vi "Initialize.vi"(0 "NI Build Specification_LV in":refnum<class "NI Build Specification_LV.lvclass">) -> (4 "NI Build Specification_LV out":refnum<class "NI Build Specification_LV.lvclass">)   [LabVIEW 2017, in "CL_G3_VIComponentBuilder.lvlib" / "NI Build Specification_LV.lvclass"]
doc: "Responsible for determining the Unique Name, Product Name, and Export's Build Specification file."
uses:
  NI Build Specification_LV.lvclass
  C:/builds/Component BuilderBT/SrcDist/Exports/Exports/Export.lvclass
  Exports/Export.lvclass/Export.ctl
  NI Build Specification_LV.lvclass/NI Build Specification_LV.ctl
  Accessors/Read Display Name XML Prop Name.vi
  Accessors/Read Unique Name XML Prop Name.vi
  Exports/Accessors/Write Export Operation Errors.vi
  Exports/Accessors/Read Export Build Specification.vi
  <vilib>/xml/Close Reference(Node).vi
  Exports/Accessors/Write Product Name.vi
  Exports/Accessors/Write unique Name.vi
  Exports/Export.lvclass
  <resource>/objmgr/DOMUserDefRef.rc
  <vilib>/xml/NI_XML.lvlib
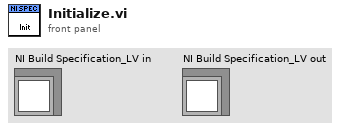
[diagram p1: front panel]
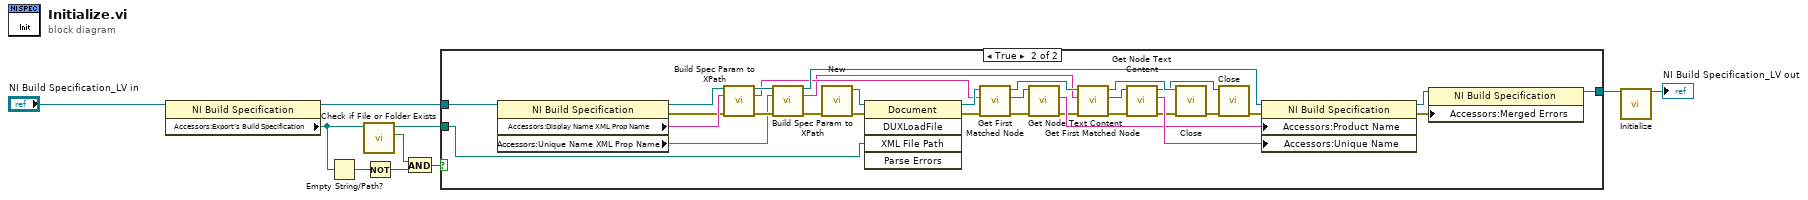
[diagram p0: block diagram]
diagram:
  n1 = property class="NI Build Specification"(reference="NI Build Specification_LV in") -> (reference out=w9:refnum<class "NI Build Specification_LV.lvclass">, "Accessors:Export's Build Specification"=w3:path)  [unwired: 1 in, 1 out]
  n2 = Empty String/Path?(string/path=w3) -> (empty?=w8:bool)
  n3 = call <vilib>:"Check if File or Folder Exists.vi"("path"=w3) -> ("file or folder exists?"=w7:bool, "dup path"=w5:path)  [unwired: 8 in, 1 out]
  n4 = Not(x=w8) -> (.not. x?=w6:bool)
  n5 = And(x=w7, y=w6) -> (x .and. y?=w4:bool)
  n6 = case shown="True" w4 {
    tunnel: w9 -> [w11 w25]
    tunnel: [w11 w40] -> w2
    tunnel: w5 -> [_ w38]
    frame False {
    }
    frame True {
      n7 = property class="NI Build Specification"(reference=w25) -> (reference out=w24:refnum<class "NI Build Specification_LV.lvclass">, error out=w13:errorcluster, "Accessors:Display Name XML Prop Name"=w20:string, "Accessors:Unique Name XML Prop Name"=w19:string)  [unwired: 1 in]
      n8 = call-dynamic "Build Spec Param to XPath.vi"("NI Build Specification"=w24, "Build Spec Parameter Name"=w20, "error in (no error)"=w13) -> ("NI Build Specification"=w23:refnum<class "NI Build Specification_LV.lvclass">, "XPath to the specific build Spec Property"=w18:string, "error out"=w21:errorcluster)  [unwired: 10 in]
      n9 = call-dynamic "Build Spec Param to XPath.vi"("NI Build Specification"=w23, "Build Spec Parameter Name"=w19, "error in (no error)"=w21) -> ("NI Build Specification"=w22:refnum<class "NI Build Specification_LV.lvclass">, "XPath to the specific build Spec Property"=w17:string, "error out"=w12:errorcluster)  [unwired: 10 in]
      n10 = call <vilib>:"New.vi"("error in (no error)"=w12) -> ("error out"=w27:errorcluster, "DOM document out"=w26:refnum<k20>)  [unwired: 7 in]
      n11 = invoke class="Document" method="DUXLoadFile"(reference=w26, error in=w27, "XML File Path"=w38) -> (reference out=w28:refnum<k20>, error out=w30:errorcluster)  [unwired: 2 in, 3 out]
      n12 = call <vilib>:"Get First Matched Node.vi"("error in (no error)"=w30, "XPath expression"=w18, "node in"=w28) -> ("error out"=w31:errorcluster, "node result"=w29:refnum<k20>, "node out"=w34:refnum<k20>)  [unwired: 6 in]
      n13 = call <vilib>:"Get Node Text Content.vi"("error in (no error)"=w31, "node in"=w29) -> ("error out"=w33:errorcluster, "node text"=w41:string)  [unwired: 7 in, 1 out]
      n14 = call <vilib>:"Get First Matched Node.vi"("error in (no error)"=w33, "XPath expression"=w17, "node in"=w34) -> ("error out"=w32:errorcluster, "node result"=w35:refnum<k20>, "node out"=w36:refnum<k20>)  [unwired: 6 in]
      n15 = call <vilib>:"Get Node Text Content.vi"("error in (no error)"=w32, "node in"=w35) -> ("error out"=w37:errorcluster, "node text"=w42:string, "node out"=w16:refnum<k20>)  [unwired: 7 in]
      n16 = call-poly <vilib>:"Close.vi"("error in (no error)"=w37, "node"=w36) -> ("error out"=w15:errorcluster)  [unwired: 7 in]
      n17 = call-poly <vilib>:"Close.vi"("error in (no error)"=w15, "node"=w16) -> ("error out"=w14:errorcluster)  [unwired: 7 in]
      n18 = property class="NI Build Specification"(reference=w22, error in=w14, "Accessors:Product Name"=w41, "Accessors:Unique Name"=w42) -> (reference out=w43:refnum<class "NI Build Specification_LV.lvclass">, error out=w39:errorcluster)
      n19 = property class="NI Build Specification"(reference=w43, "Accessors:Merged Errors"=w39) -> (reference out=w40:refnum<class "NI Build Specification_LV.lvclass">)  [unwired: 1 in, 1 out]
    }
  }
  n20 = call-parent "Initialize.vi"("Export in"=w2) -> ("Export out"=→"NI Build Specification_LV out":refnum<class "NI Build Specification_LV.lvclass">)  [unwired: 14 in]
